vi "GeneratePixelWave.vi"(1 "Fs":u64, 2 "Delay between waves (us)":dbl, 3 "Waves per Pixel":u32, 4 "Single Wave":u16[](array[numeric])) -> (0 "Pixel Wave":cluster{dbl[], "R":dbl[]})   [LabVIEW 2018]
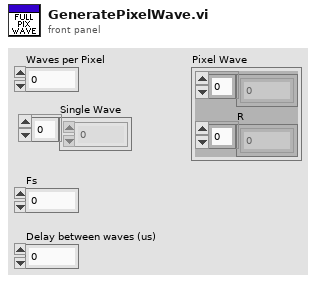
[diagram p1: front panel]
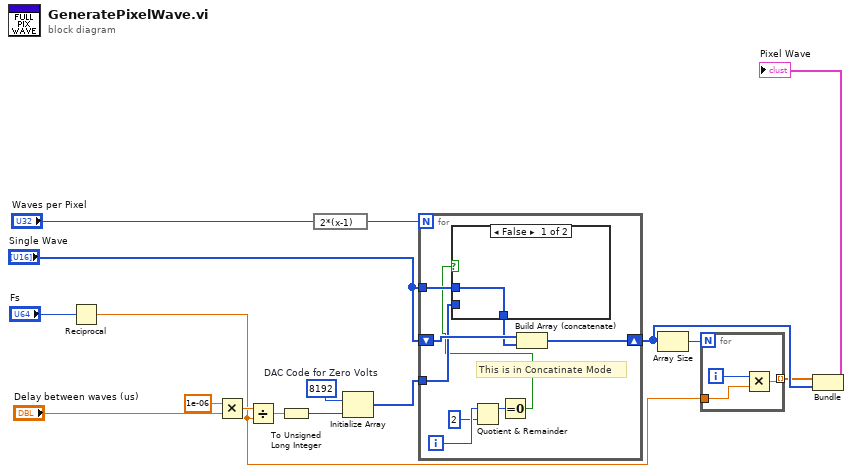
[diagram p0: block diagram]
diagram:
  w1 = 8192  # DAC Code for Zero Volts
  n1 = Reciprocal(x="Fs") -> (1/x=w2:dbl)
  n2 = Multiply(x=1e-06, y="Delay between waves (us)") -> (x*y=w6:dbl)
  n3 = Divide(x=w6, y=w2) -> (x/y=w4:dbl)
  n4 = To Unsigned Long Integer(number=w4) -> (unsigned 32bit integer=w5:u32)
  n5 = expression code="2*(x-1)"("Waves per Pixel") -> (w9:u32)
  n6 = Initialize Array(w1, w5) -> (w10:i32[])
  n7 = for {
    N: w9 -> [_]
    tunnel: w10 -> [w22]
    tunnel: "Single Wave" -> [w23]
    shift-right: [w17] -> w15
    shift-left: "Single Wave" -> [w25]
    i -> [w21]
    # "This is in Concatinate Mode"
    n8 = Quotient & Remainder(x=w21, y=2) -> (x-y*floor(x/y)=w19:i32)  [unwired: 1 out]
    n9 = Equal To 0?(x=w19) -> (x = 0?=w18:bool)
    n10 = case shown="False" w18 {
      tunnel: [w26 w27] -> w24
      tunnel: w23 -> [w26 _]
      tunnel: w22 -> [_ w27]
      frame False {
      }
      frame True {
      }
    }
    n11 = Build Array (concatenate)(w25, w24) -> (w17:i32[])
  }
  n12 = Array Size(array=w15) -> (size(s)=w12:i32)
  n13 = for {
    N: w12 -> [_]
    tunnel: [w29] -> w14 mode=indexing
    tunnel: w2 -> [w28]
    i -> [w30]
    n14 = Multiply(x=w30, y=w28) -> (x*y=w29:dbl)
  }
  n15 = Bundle(w14, "Single Wave"=w15) -> (→"Pixel Wave":cluster{dbl[], "Single Wave":i32[]})  [unwired: 1 in]
